vi "Read Waveform Measurement (Standard).vi"(0 "VISA resource name":refnum<visa-resource-name>, 5 "Source (0: Channel 1)":u16(ring) items=["Channel 1", "Channel 2", "Channel 3", "Channel 4", "Memory 1", "Memory 2", "Memory 3", "Memory 4", "Function 1", "Function 2", "Function 3", "Function 4", "Function 5", "Function 6", "Function 7", "Function 8", "Other"], 7 "Custom Source ID":string, 9 "Measurement (0: Amplitude)":u16(ring) items=["Amplitude", "Area", "Base", "Cycles", "Delay", "Duration", "Duty Cycle *", "Fall Time (90-10) *", "Fall Time (80-20) *", "First", "Frequency *", "Last", "Maximum", "Mean", "Median", "Minimum", "Num Points", "Overshoot (Negative) *", "Overshoot (Positive) *", "Peak-Peak", "Period *", "Risetime (10-90) *", "Risetime (20-80) *", "RMS", "Standard Deviation", "Top", "Width (Negative slope) *", "Width (Positve slope)"], 11 "error in (no error)":errorcluster) -> (4 "VISA resource name out":refnum<visa-resource-name>, 6 "Value":dbl, 8 "Status":string, 15 "error out":errorcluster)   [LabVIEW 2015, in "LeCroy Wave Series.lvlib"]
doc: "This VI returns a the result of the requested measurement. Note that not all parameters are available on all scopes! (The VI will return an \"unresolved parsing error\" if an unsupported measurement is requested)\n\nThe measurements that you can select in this VI do not require arguments such as reference levels, slopes, etc; for parameters that require \"arguments\" configure them on the scope, and readout the result with the VI \"Read Px Measurement.vi\"\n\nNote that most \"horizontal\" parameters (e.g. parameters that return a time or frequency) are multi-valued. For these parameters, the last occurence is returned, as opposed to the average value over the entire sweep."
uses:
  <instrlib>/LeCroy Wave Series/LeCroy Wave Series.lvlib
panel:
  # "Note for functions with a *: The last measured value is returned by these functions, and not the average value  over the sweep. See VI help for more information."
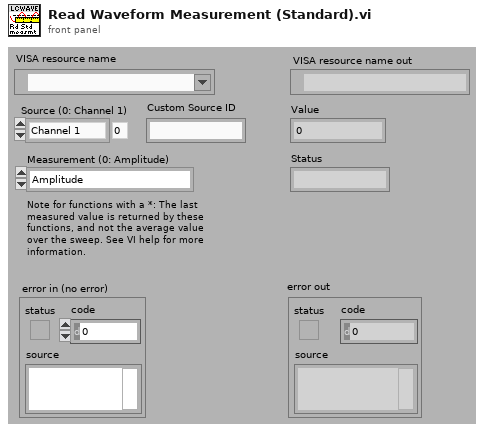
[diagram p1: front panel]
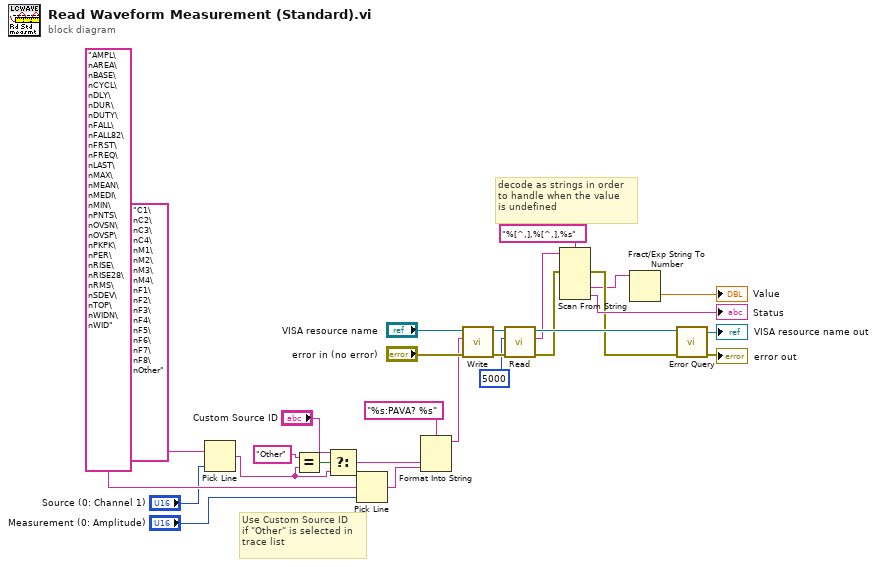
[diagram p0: block diagram]
diagram:
  # "Use Custom Source ID\nif \"Other\" is selected in \ntrace list"
  # "decode as strings in order \nto handle when the value\nis undefined"
  n1 = Pick Line(multi-line string="C1\nC2\nC3\nC4\nM1\nM2\nM3\nM4\nF1\nF2\nF3\nF4\nF5\nF6\nF7\nF8\nOther", line index="Source (0: Channel 1)") -> (output string=w10:string)  [unwired: 1 in]
  n2 = Equal?(x="Other", y=w10) -> (x = y?=w12:bool)
  n3 = Select(t="Custom Source ID", s=w12, f=w10) -> (s? t:f=w8:string)
  n4 = Pick Line(multi-line string="AMPL\nAREA\nBASE\nCYCL\nDLY\nDUR\nDUTY\nFALL\nFALL82\nFRST\nFREQ\nLAST\nMAX\nMEAN\nMEDI\nMIN\nPNTS\nOVSN\nOVSP\nPKPK\nPER\nRISE\nRISE28\nRMS\nSDEV\nTOP\nWIDN\nWID", line index="Measurement (0: Amplitude)") -> (output string=w23:string)  [unwired: 1 in]
  n5 = Format Into String(format string="%s:PAVA? %s", w8, w23) -> (resulting string=w15:string)  [unwired: 2 in, 1 out]
  n6 = call <instrlib>:"Write.vi"("error in (no error)"="error in (no error)", "Write Buffer"=w15, "VISA resource name"="VISA resource name") -> ("error out"=w20:errorcluster, "VISA resource name out"=w21:refnum<visa-resource-name>)  [unwired: 6 in, 1 out]
  n7 = call <instrlib>:"Read.vi"("error in (no error)"=w20, "Byte Count"=u32 5000, "VISA resource name"=w21) -> ("error out"=w6:errorcluster, "Read Buffer"=w7:string, "VISA resource name out"=w18:refnum<visa-resource-name>)  [unwired: 5 in, 1 out]
  n8 = Scan From String(format string="%[^,],%[^,],%s", input string=w7, error in=w6) -> (error out=w4:errorcluster, output 2=w2:string, output 3=→"Status":string)  [unwired: 5 in, 2 out]
  n9 = Fract/Exp String To Number(string=w2) -> (number=→"Value":dbl)  [unwired: 3 in, 1 out]
  n10 = call <instrlib>:"Error Query.vi"("error in (no error)"=w4, "VISA resource name"=w18) -> ("error out"=→"error out":errorcluster, "VISA resource name out"=→"VISA resource name out":refnum<visa-resource-name>)  [unwired: 6 in, 2 out]
